vi "LIndex.vi"(0 "reference in":refnum<class "Redis.lvclass">, 1 "Key":string, 7 "Index":string, 11 "Error In":errorcluster) -> (4 "reference out":refnum<class "Redis.lvclass">, 8 "Data":T1, 15 "Error Out":errorcluster)   [LabVIEW 2020, in "Redis.lvclass"]
doc: "Returns the element at index index in the list stored at key. The index is zero-based, so 0 means the first element, 1 the second element and so on. Negative indices can be used to designate elements starting at the tail of the list. Here, -1 means the last element, -2 means the penultimate and so forth."
uses:
  Redis.lvclass
  RedisDataType.ctl
  ReplyDataTypeEnum.ctl
  Redis.lvclass/Redis.ctl
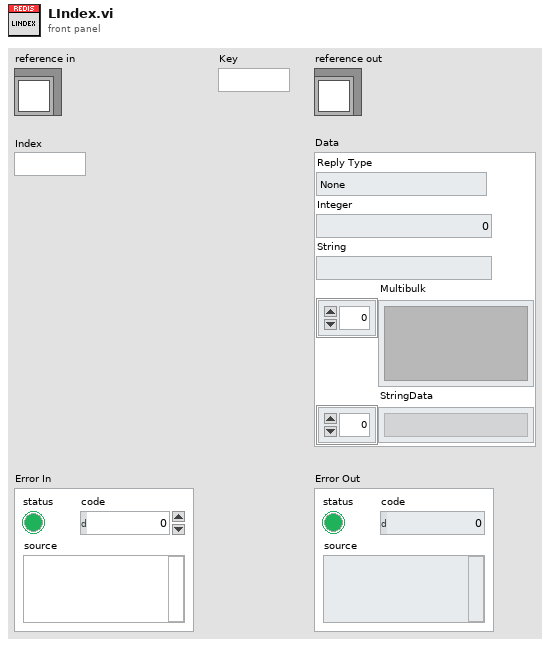
[diagram p1: front panel]
types:
  T1 = typedef "Redis.lvclass/RedisDataType.ctl" = cluster{"Reply Type":T2, "Integer":i64, "String":string, "Multibulk":variant[], "StringData":string[]}
  T2 = typedef "Redis.lvclass/ReplyDataTypeEnum.ctl" = enum16{"None", "Error", "Status", "Nil", "Integer", "String", "Multibulk"}
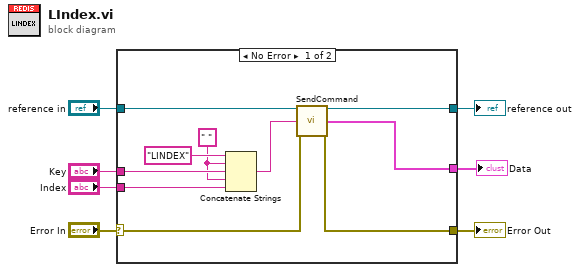
[diagram p0: block diagram]
diagram:
  n1 = case shown="No Error" "Error In" {
    selector: "Error In" -> [w15 w19]
    tunnel: [w14 w19] -> w6
    tunnel: [w17 w18] -> w4
    tunnel: "reference in" -> [w16 w18]
    tunnel: [w13 _] -> w3
    tunnel: "Key" -> [w11 _]
    tunnel: "Index" -> [w8 _]
    frame No Error {
      w9 = " "
      n2 = Concatenate Strings("LINDEX", w9, w11, w9, w8) -> (w10:string)
      n3 = call "SendCommand.vi"("reference in"=w16, "Command"=w10, "Error In"=w15) -> ("reference out"=w17:refnum<class "Redis.lvclass">, "Data"=w13:T1, "Error Out"=w14:errorcluster)  [unwired: 10 in]
    }
    frame Error {
    }
  }
  "Error Out" <- w6
  "reference out" <- w4
  "Data" <- w3
